vi "leak_tester_0.vi"() -> ()   [LabVIEW 2020]
uses:
  event_controller.ctl
  <vilib>/Spiers New Technologies/SNT/Alfred-Connector/Utilities/Parse Item Label Data Output.ctl
  <vilib>/Spiers New Technologies/SNT/Alfred-Connector/Alfred.lvlib
panel:
  in  "LOGOUT":bool
  in  "submission":bool
  in  "RETURN":bool
  in  "test":bool
  out "Parse Item Label Data out":T1
  in  "Barcode":string="IID:287454SN:CM5810B759GBRED11031550695872PN:CM5810B759GBEND"
  out "User ID":string
  out "Current State":T2
  in  "Badge":string="3B 88 01 00 03 08 06 66 00 77 80 78"
  in  "enter":bool
  in  "stop":bool
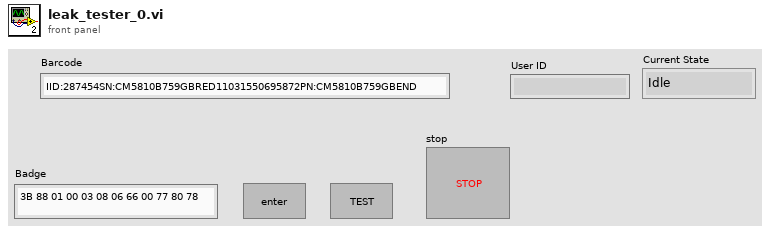
[diagram p1: front panel]
types:
  T1 = typedef "Alfred.lvlib/Parse Item Label Data Output.ctl" = cluster{"qr_code":string, "serial_number":string, "part_number":string, "item_id":string, "item_type_id":string, "item_type":string, "status":string, "status_id":string, "business_unit":string, "generation":string, "section":string, "chemistry_type":string, "human_description":string, "location_allowed":string, "business_unit_id":string, "previously_recertified":string, "capacity":string, "capacity_color_code":string, "soc_30_percent_voltage":string, "model_year":string, "pack_item_id":string, "error_message":string}
  T2 = typedef "event_controller.ctl" = enum16{"Idle", "LoginFalse", "BatteryScan", "BatteryError", "Testing", "Submission"}
  T3 = cluster{"item_id":string, "item_type_id":string, string}
  T4 = cluster{"Username":string, "Badge":string, "Username":string, "Privilege":string}
  T5 = typedef "Alfred.lvlib/Login Info Return.ctl" = cluster{"User ID":string, "Username":string, "First Name":string, "Last Name":string, "E-mail":string, "Time Zone":string, "Error Message":string}
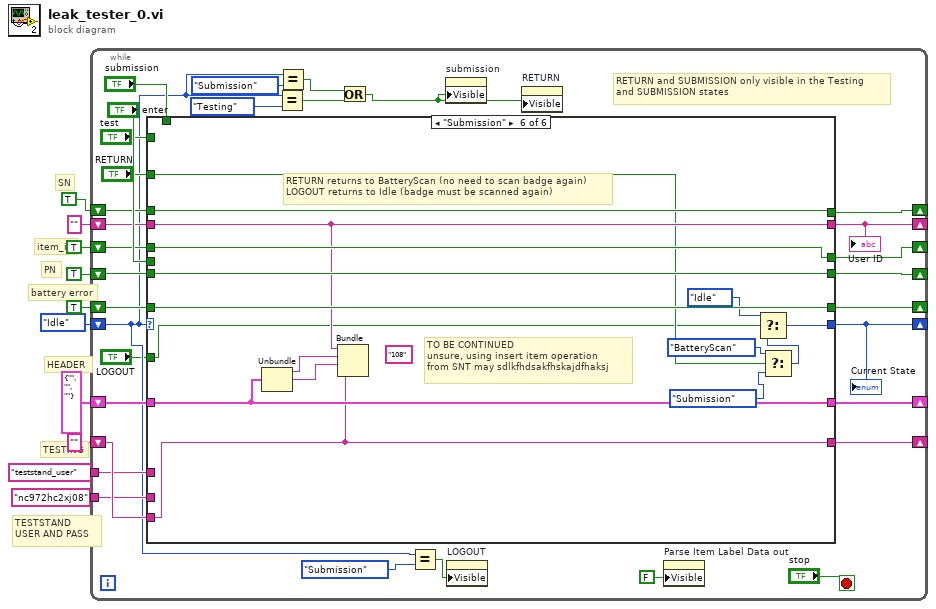
[diagram p0: block diagram]
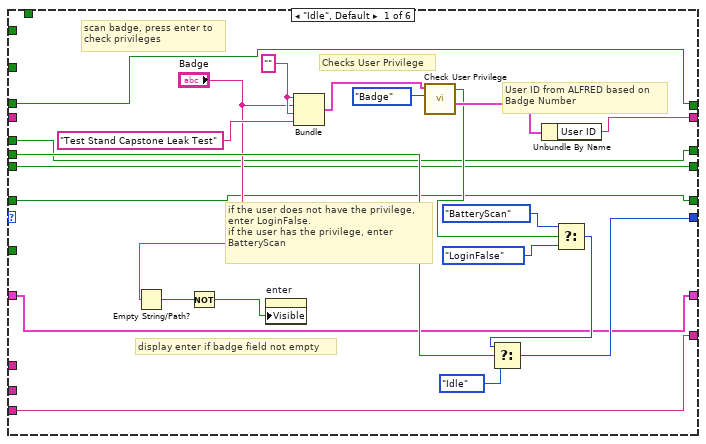
[diagram p2: hidden frame]
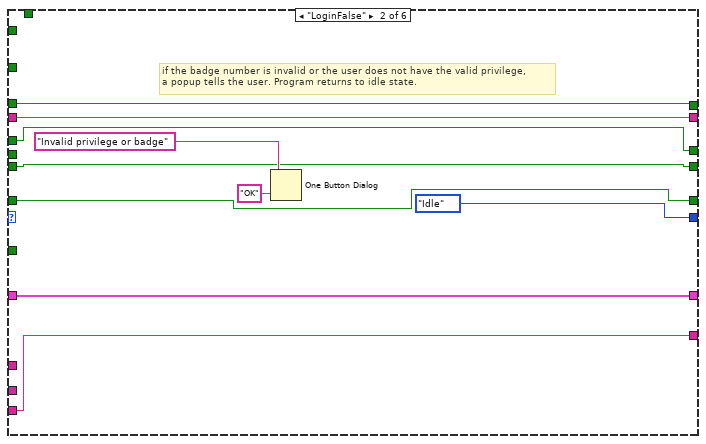
[diagram p3: hidden frame]
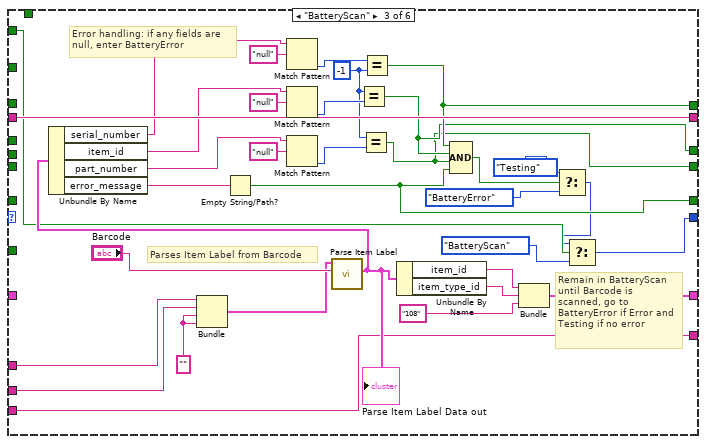
[diagram p4: hidden frame]
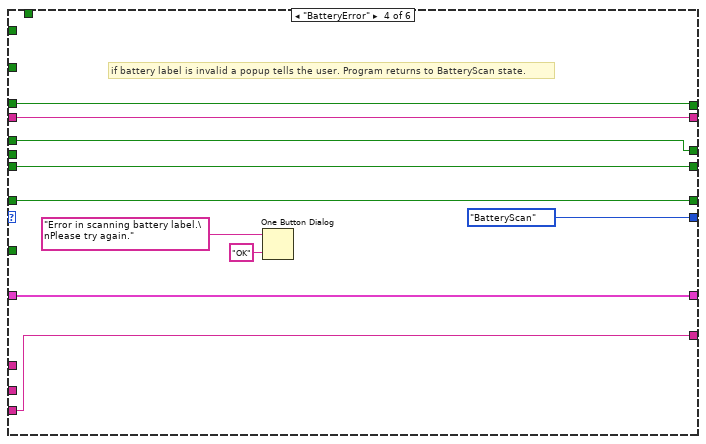
[diagram p5: hidden frame]
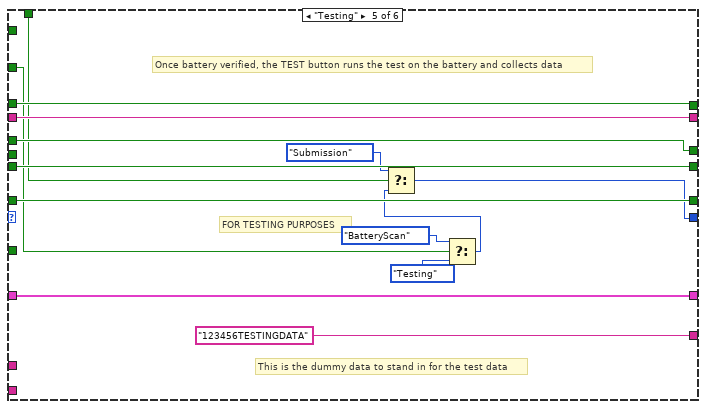
[diagram p6: hidden frame]
diagram:
  # "TESTSTAND\nUSER AND PASS"
  # "HEADER"
  # "TESTING"
  # "battery error"
  # "PN"
  # "item_id"
  # "SN"
  n1 = while {
    shift-right: [w41] -> _
    shift-left: event_controller."Idle" -> [w14]
    shift-right: [w39] -> _
    shift-left: "" ("User ID") -> [w38]
    shift-right: [w37] -> _
    shift-left: T3 {"item_id"="", "item_type_id"="", ""} -> [w36]
    shift-right: [w35] -> _
    shift-left: TRUE -> [w34]
    shift-right: [w33] -> _
    shift-left: TRUE -> [w30]
    shift-right: [w32] -> _
    shift-left: TRUE -> [w29]
    shift-right: [w31] -> _
    shift-left: TRUE -> [w28]
    shift-right: [w24] -> _
    shift-left: "" -> [w23]
    tunnel: "teststand_user" -> [w16]
    tunnel: "nc972hc2xj08" -> [w15]
    stop <- "stop" stop-if-true
    # "RETURN and SUBMISSION only visible in the Testing\nand SUBMISSION states"
    n2 = case shown="\"Submission\"" w14 {
      tunnel: [w55 event_controller."Idle" w78 event_controller."BatteryScan" w120 w133] -> w41
      tunnel: "enter" -> [w56 _ _ _ _ _]
      tunnel: [w52 w71 w108 w118 w132 w144] -> w39
      tunnel: w38 -> [_ w71 w108 w118 w132 w144]
      tunnel: [w48 w70 w101 w117 w131 w143] -> w37
      tunnel: w36 -> [w48 w70 _ w117 w131 w143]
      tunnel: [w47 w69 w85 w116 w130 w148] -> w35
      tunnel: w34 -> [w47 w69 _ w116 w130 w148]
      tunnel: [w46 w68 w84 w115 w129 w147] -> w33
      tunnel: [w45 w67 w83 w114 w128 w146] -> w32
      tunnel: [w44 w66 w82 w113 w127 w145] -> w31
      tunnel: w30 -> [w46 w68 _ w115 w129 w147]
      tunnel: w29 -> [w45 w67 _ w114 w128 w146]
      tunnel: w28 -> [w44 w66 _ w113 w127 w145]
      tunnel: "test" -> [_ _ w81 _ _ _]
      tunnel: "RETURN" -> [_ _ _ _ w126 w139]
      tunnel: [w43 w65 w77 w109 "123456TESTINGDATA" w140] -> w24
      tunnel: w23 -> [w43 w65 w77 w109 _ w140]
      tunnel: "submission" -> [_ _ _ _ w119 _]
      tunnel: w16 -> [_ _ w76 _ _ _]
      tunnel: w15 -> [_ _ w75 _ _ _]
      tunnel: "LOGOUT" -> [_ _ _ _ _ w136]
      frame "Idle", Default {
        w62 = "" ("Username")
        # "display enter if badge field not empty"
        # "if the user does not have the privilege, \nenter LoginFalse. \nif the user has the privilege, enter \nBatteryScan"
        # "User ID from ALFRED based on\nBadge Number"
        # "Checks User Privilege"
        # "scan badge, press enter to \ncheck privileges"
        n3 = Empty String/Path?(string/path="Badge") -> (empty?=w50:bool)
        n4 = Not(x=w50) -> (.not. x?=w49:bool)
        n5 = property on="enter" class="Bool"("Visible"=w49) -> ()  [unwired: 2 in, 2 out]
        n6 = Bundle("Username"=w62, "Badge"="Badge", "Username"=w62, "Privilege"="Test Stand Capstone Leak Test") -> (w60:T4)  [unwired: 1 in]
        n7 = call <vilib>:"Check User Privilege.vi"("Login Method"=enum16{"User ID/PW", "Badge"}."Badge", "Login Data Input"=w60) -> ("Login Info"=w63:T5, "Valid?"=w53:bool)  [unwired: 7 in, 1 out]
        n8 = Unbundle By Name(w63) -> ("User ID"=w52:string)
        n9 = Select(t=event_controller."BatteryScan", s=w53, f=event_controller."LoginFalse") -> (s? t:f=w54:T2)
        n10 = Select(t=w54, s=w56, f=event_controller."Idle") -> (s? t:f=w55:T2)
      }
      frame "LoginFalse" {
        # "if the badge number is invalid or the user does not have the valid privilege,\na popup tells the user. Program returns to idle state."
        n11 = One Button Dialog(message="Invalid privilege or badge", button name ("OK")="OK") -> ()  [unwired: 1 out]
      }
      frame "BatteryScan" {
        w91 = -1 ("y")
        w105 = ""
        # "Remain in BatteryScan\nuntil Barcode is \nscanned, go to \nBatteryError if Error and\nTesting if no error"
        # "Error handling: if any fields are \nnull, enter BatteryError"
        # "Parses Item Label from Barcode"
        n12 = Bundle(w76, w75, w105, w105) -> (w106:cluster{string, string, string, string})  [unwired: 1 in]
        n13 = call <vilib>:"Parse Item Label.vi"("Barcode"="Barcode", "Alfred Data"=w106) -> ("Parse Item Label Data out"=w100:T1)  [unwired: 6 in, 3 out]
        "Parse Item Label Data out" <- w100
        n14 = Unbundle By Name(w100) -> ("serial_number"=w96:string, "item_id"=w95:string, "part_number"=w94:string, "error_message"=w89:string)
        n15 = Empty String/Path?(string/path=w89) -> (empty?=w82:bool)
        n16 = Match Pattern(string=w96, regular expression="null") -> (offset past match=w93:i32)  [unwired: 1 in, 3 out]
        n17 = Match Pattern(string=w95, regular expression="null") -> (offset past match=w92:i32)  [unwired: 1 in, 3 out]
        n18 = Match Pattern(string=w94, regular expression="null") -> (offset past match=w90:i32)  [unwired: 1 in, 3 out]
        n19 = Equal?(x=w91, y=w92) -> (x = y?=w84:bool)
        n20 = Equal?(x=w91, y=w90) -> (x = y?=w83:bool)
        n21 = Equal?(x=w93, y=w91) -> (x = y?=w85:bool)
        n22 = Unbundle By Name(w100) -> ("item_id"=w104:string, "item_type_id"=w103:string)
        n23 = Compound Arithmetic op=AND(w85, w84, w83, w82) -> (w88:bool)
        n24 = Bundle("item_id"=w104, "item_type_id"=w103, "108") -> (w101:T3)  [unwired: 1 in]
        n25 = Select(t=event_controller."Testing", s=w88, f=event_controller."BatteryError") -> (s? t:f=w79:T2)
        n26 = Select(t=w79, s=w81, f=event_controller."BatteryScan") -> (s? t:f=w78:T2)
      }
      frame "BatteryError" {
        # "if battery label is invalid a popup tells the user. Program returns to BatteryScan state."
        n27 = One Button Dialog(message="Error in scanning battery label.\nPlease try again.", button name ("OK")="OK") -> ()  [unwired: 1 out]
      }
      frame "Testing" {
        # "This is the dummy data to stand in for the test data"
        # "Once battery verified, the TEST button runs the test on the battery and collects data"
        # "FOR TESTING PURPOSES"
        n28 = Select(t=event_controller."BatteryScan", s=w126, f=event_controller."Testing") -> (s? t:f=w121:T2)
        n29 = Select(t=event_controller."Submission", s=w119, f=w121) -> (s? t:f=w120:T2)
      }
      frame "Submission" {
        (unwired) "108" ("Item Operation ID")
        # "RETURN returns to BatteryScan (no need to scan badge again)\nLOGOUT returns to Idle (badge must be scanned again)"
        # "TO BE CONTINUED\nunsure, using insert item operation\nfrom SNT may sdlkfhdsakfhskajdfhaksj"
        n30 = Unbundle(w143) -> ("item_id"=w142:string, "item_type_id"=w141:string)  [unwired: 1 out]
        n31 = Bundle("User ID"=w144, "item_id"=w142, "item_type_id"=w141, w140) -> ()  [unwired: 1 in, 1 out]
        n32 = Select(t=event_controller."BatteryScan", s=w139, f=event_controller."Submission") -> (s? t:f=w134:T2)
        n33 = Select(t=event_controller."Idle", s=w136, f=w134) -> (s? t:f=w133:T2)
      }
    }
    "Current State" <- w41
    "User ID" <- w39
    n34 = Equal?(x=w14, y=event_controller."Testing") -> (x = y?=w20:bool)
    n35 = Equal?(x=w14, y=event_controller."Submission") -> (x = y?=w17:bool)
    n36 = Or(x=w17, y=w20) -> (x .or. y?=w19:bool)
    n37 = Equal?(x=w14, y=event_controller."Submission") -> (x = y?=w13:bool)
    n38 = property on="submission" class="Bool"("Visible"=w19) -> ()  [unwired: 2 in, 2 out]
    n39 = property on="LOGOUT" class="Bool"("Visible"=w13) -> ()  [unwired: 2 in, 2 out]
    n40 = property on="RETURN" class="Bool"("Visible"=w19) -> ()  [unwired: 2 in, 2 out]
    n41 = property on="Parse Item Label Data out" class="Clust (strict)"("Visible"=FALSE) -> ()  [unwired: 2 in, 2 out]
  }
